vi "Test Pre-filter.vi"(8 "error in (no error)":errorcluster, 11 "Lockin.DAQ in":refnum<class "Instrument.DAQ.lvclass">) -> (0 "error out":errorcluster, 3 "Lockin.DAQ out":refnum<class "Instrument.DAQ.lvclass">)   [LabVIEW 2019, in "Instrument.Lockin.lvlib" / "Instrument.DAQ.lvclass"]
uses:
  Instrument.DAQ.lvclass
  DAQmx/DAQmx.lvclass
  C:/Program Files/National Instruments/LabVIEW 2019/vi.lib/JKI/JKI SMO/SMO/SMO.lvclass
  Typedefs/AO.Channel.Function--Enum.ctl
  Typedefs/AO.Channel--Cluster--Array.ctl
  Typedefs/REF.Channel--Cluster--Array.ctl
  Typedefs/DAQ.Sampling.Sampling--Cluster.ctl
  Typedefs/AO.Channel--Cluster.ctl
  Typedefs/REF.Channel--Cluster.ctl
  Typedefs/AI.Channel--Cluster.ctl
  Typedefs/AI.Channel--Cluster--Array.ctl
  Typedefs/Configuration.Prefilter--Cluster.ctl
panel:
  out "x-y":dbl(graph)
  in  "Configuration.Prefilter":T1
  out "appended array":waveform(dbl)[](array[waveform])
  out "Waveform Graph":waveform(dbl)[](graph)
  in  "AI Channels":T2 {"reference index" min=1; "References" items=["", "1", "2", "3", "4", "5", "6", "7", "8", "9"]; "Channel" min=1}
  in  "REF Channels":T4 {"Roll-Off" min=1 max=4; "TC" min=1e-06 max=100.0 format="%#_3p"; "Phase" format="%#_3p"; "Frequency" min=1e-06 max=102400.0 format="%#_6p"; "Channel" min=1}
  in  "sampling":T6={"Fs"=204789.0, "#s"=15753} {"Fs" format="%#_13g"}
  in  "stop":bool
  in  "AO Channels":T7=[{"Enable?"=FALSE, "Channel"=0, "Amplitude"=0.0, "Offset"=0.0, "Frequency"=0.1, "Phase"=0.0, "Function"=enum."sine", "Sweeping?"=FALSE, "Limit AC"=FALSE, "Limit DC?"=FALSE, "Duty Cycle"=FALSE}] {"Phase" format="%#_3g"; "Frequency" min=0.0001 max=200000.0 format="%#_6p"; "Offset" format="%#_6p"; "Amplitude" min=0.0 max=10.0 format="%#_6p"}
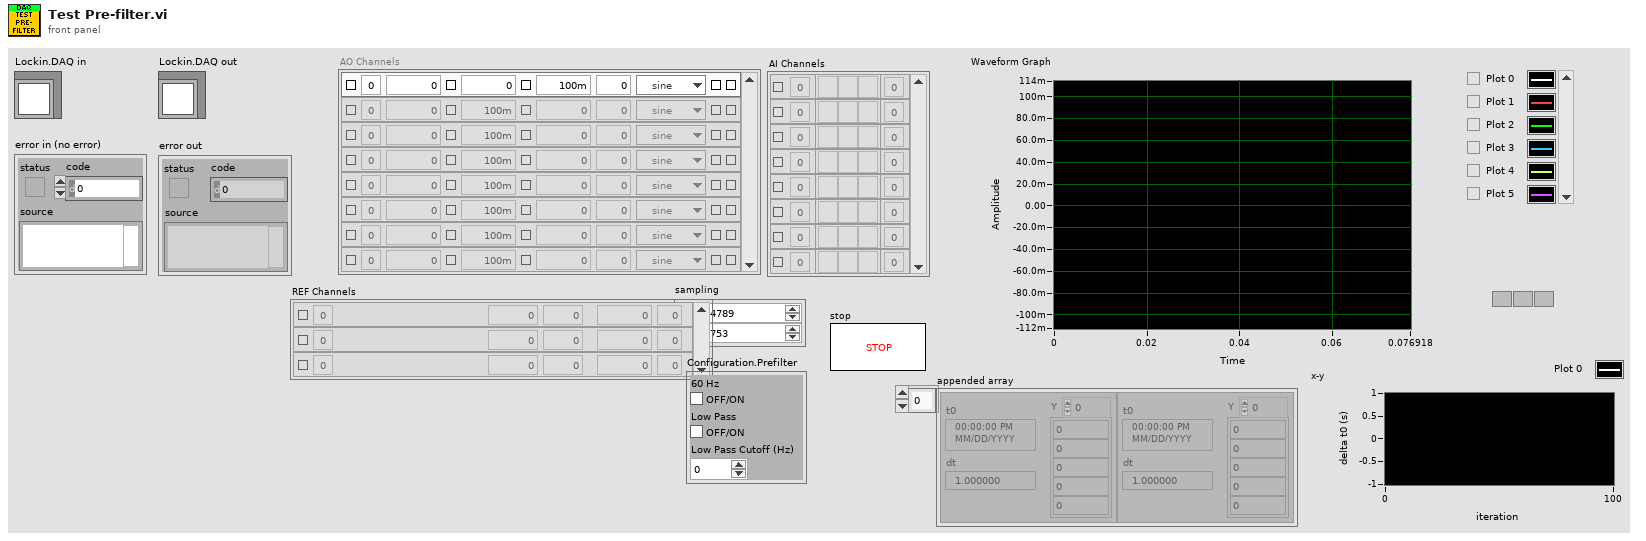
[diagram p1: front panel]
types:
  T1 = typedef "Instrument.Lockin.lvlib/Instrument.DAQ.lvclass/Configuration.Prefilter--Cluster.ctl" = cluster{"60 Hz":bool, "Low Pass":bool, "Low Pass Cutoff (Hz)":dbl}
  T2 = typedef "Instrument.Lockin.lvlib/Instrument.DAQ.lvclass/AI.Channel--Cluster--Array.ctl" = T3[]
  T3 = typedef "Instrument.Lockin.lvlib/Instrument.DAQ.lvclass/AI.Channel--Cluster.ctl" = cluster{"Enable?":bool, "Channel":i32, "References":u16[], "reference index":i32}
  T4 = typedef "Instrument.Lockin.lvlib/Instrument.DAQ.lvclass/REF.Channel--Cluster--Array.ctl" = T5[]
  T5 = typedef "Instrument.Lockin.lvlib/Instrument.DAQ.lvclass/REF.Channel--Cluster.ctl" = cluster{"Enable?":bool, "Channel":i32, "Frequency":dbl, "Phase":dbl, "TC":dbl, "Roll-Off":i32}
  T6 = typedef "Instrument.Lockin.lvlib/Instrument.DAQ.lvclass/DAQ.Sampling.Sampling--Cluster.ctl" = cluster{"Fs":dbl, "#s":i32}
  T7 = typedef "Instrument.Lockin.lvlib/Instrument.DAQ.lvclass/AO.Channel--Cluster--Array.ctl" = T8[]
  T8 = typedef "Instrument.Lockin.lvlib/Instrument.DAQ.lvclass/AO.Channel--Cluster.ctl" = cluster{"Enable?":bool, "Channel":i32, "Amplitude":dbl, "Offset":dbl, "Frequency":dbl, "Phase":dbl, "Function":T9, "Sweeping?":bool, "Limit AC":bool, "Limit DC?":bool, "Duty Cycle":bool}
  T9 = typedef "Instrument.Lockin.lvlib/Instrument.DAQ.lvclass/AO.Channel.Function--Enum.ctl" = enum16{"sine", "square", "triangle", "saw"}
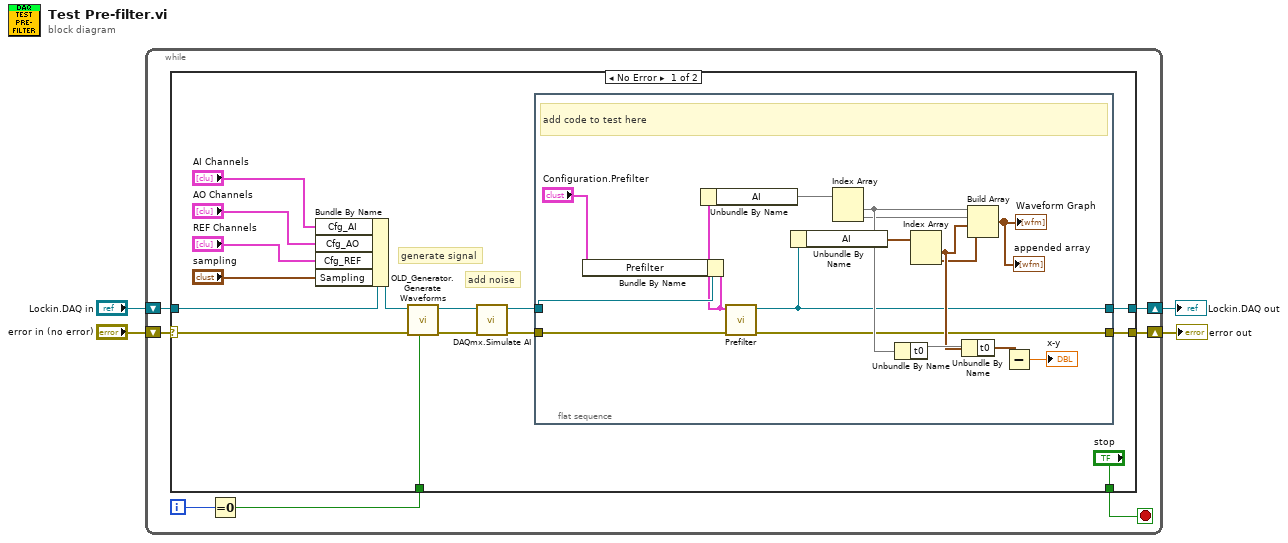
[diagram p0: block diagram]
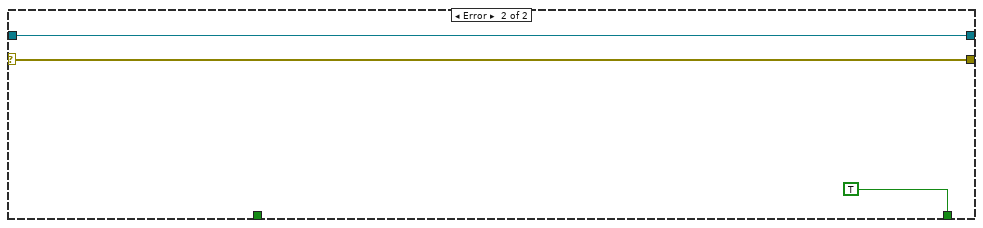
[diagram p2: hidden frame]
diagram:
  n1 = while {
    shift-right: [w10] -> w3
    shift-left: "error in (no error)" -> [w11]
    shift-right: [w8] -> w1
    shift-left: "Lockin.DAQ in" -> [w9]
    i -> [w6]
    stop <- w5 stop-if-true
    n2 = Equal To 0?(x=w6) -> (x = 0?=w7:bool)
    n3 = case shown="No Error" w11 {
      selector: w11 -> [w25 w45]
      tunnel: [w22 w45] -> w10
      tunnel: [w24 w44] -> w8
      tunnel: w9 -> [w13 w44]
      tunnel: w7 -> [w21 _]
      tunnel: ["stop" TRUE ("stop")] -> w5
      frame No Error {
        # "generate signal"
        # "add noise"
        n4 = Bundle By Name(cluster=w13, "Cfg_AI"="AI Channels", "Cfg_AO"="AO Channels", "Cfg_REF"="REF Channels", "Sampling"="sampling") -> (w12:refnum<class "Instrument.DAQ.lvclass">)
        n5 = call "OLD_Generator.Generate Waveforms.vi"("reset phase?"=w21, "error in (no error)"=w25, "Instrument.DAQ"=w12) -> ("error out"=w26:errorcluster, "Instrument.DAQ"=w14:refnum<class "Instrument.DAQ.lvclass">)  [unwired: 6 in, 1 out]
        n6 = call "DAQmx.Simulate AI.vi"("error in (no error)"=w26, "DAQmx in"=w14) -> ("error out"=w23:errorcluster, "DAQmx out"=w15:refnum<class "DAQmx.lvclass">)  [unwired: 6 in, 2 out]
        n7 = flat-sequence {
          tunnel: [w28] -> w24
          tunnel: w23 -> [w29]
          tunnel: [w27] -> w22
          tunnel: w15 -> [w31]
          frame #0 {
            # "add code to test here"
            n8 = Bundle By Name(cluster=w31, "Prefilter"="Configuration.Prefilter") -> (w30:cluster{})
            n9 = Unbundle By Name(w30) -> ("AI"=w40)
            n10 = call "Prefilter.vi"("error in (no error)"=w29, "Instrument.DAQ in"=w30) -> ("error out"=w27:errorcluster, "Instrument.DAQ out"=w28:refnum<class "Instrument.DAQ.lvclass">)  [unwired: 7 in, 1 out]
            n11 = Unbundle By Name(w28) -> ("AI"=w39:waveform(dbl)[])
            n12 = Index Array(array=w40) -> (element #1=w33, element #2=w32)  [unwired: 2 in]
            n13 = Unbundle By Name(w33) -> ("t0"=w36)
            n14 = Index Array(array=w39) -> (element #1=w35:waveform(dbl), element #2=w34:waveform(dbl))  [unwired: 2 in]
            n15 = Unbundle By Name(w35) -> ("t0"=w37:timestamp)
            n16 = Build Array(w33, w32, w35, w34) -> (→"Waveform Graph" →"appended array":waveform(dbl)[])
            n17 = Subtract(x=w37, y=w36) -> (x-y=→"x-y":dbl)
          }
        }
      }
      frame Error {
      }
    }
  }
  "error out" <- w3
  "Lockin.DAQ out" <- w1
